vi "Stop Core.vi"(10 "final error code":i32, 11 "Trace Controller in":refnum<class "Trace Controller.lvclass">) -> (3 "Trace Controller out":refnum<class "Trace Controller.lvclass">)   [LabVIEW 2014, in "Robot Actor Framework.lvlib" / "Trace.lvlib" / "Trace Controller.lvclass"]
doc: "(<B>Filename</B>: Actor Framework.lvlib:Actor.lvclass:Stop Core.vi)\n\nDefines what the actor does before it stops. Use the <B>final error code</B> input to determine whether the actor shut down in response to an error.\n\nBy default, this method does nothing. A descendant class may override it to define behavior, such as shutting down any processes the actor initiated in its override of the Actor Core method."
uses:
  Trace Controller.lvclass
  Trace Controller.lvclass/Trace Controller.ctl
  System Actor/System Actor Class/System Actor.lvclass
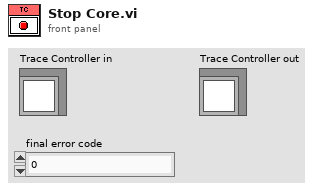
[diagram p1: front panel]
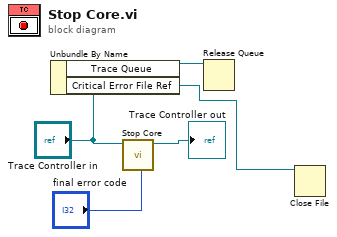
[diagram p0: block diagram]
diagram:
  n1 = Unbundle By Name("Trace Controller in") -> ("Trace Queue"=w2:refnum<queue>, "Critical Error File Ref"=w1:refnum<file>)
  n2 = call-parent "Stop Core.vi"("final error code"="final error code", "System Actor in"="Trace Controller in") -> ("System Actor out"=→"Trace Controller out":refnum<class "Trace Controller.lvclass">)  [unwired: 9 in]
  n3 = Release Queue(queue=w2) -> ()  [unwired: 2 in, 3 out]
  n4 = Close File(refnum=w1) -> ()  [unwired: 1 in, 2 out]
